vi "TcA02-003_ModifyingObjectAttributesMultipleTimes.vi"(1 "Input buffer":T3="1", 3 "Invocation info":T2, 5 "error in (no error)":errorcluster, 6 "Add log to result?":bool) -> (16 "Test Data":T1 {"Numeric Measurement" format="%.2f"}, 19 "error out":errorcluster)   [LabVIEW 2020]
doc: "Test case template."
uses:
  Shared/Support_InputBuffer.ctl
  Shared/Support_InvocationInfo.ctl
  Shared/Support_TestData.ctl
  TestClasses/G#SubClass2_class/G#SubClass2.lvclass
  TestClasses/G#BaseClass2_class/G#BaseClass2.lvclass
  TestClasses/G#BaseClass1_class/G#BaseClass1.lvclass
  <vilib>/addons/_AddQ/G#Object/G#Object.lvclass
panel:
  in  "Test name":string="TcA02-003 Modifying object attributes multiple times"
  out "Test result":bool
  out "Result":string
  # "Verify that object attributes can be modified\nmultiple times unaffected by other objects."
  # "Sub test case"
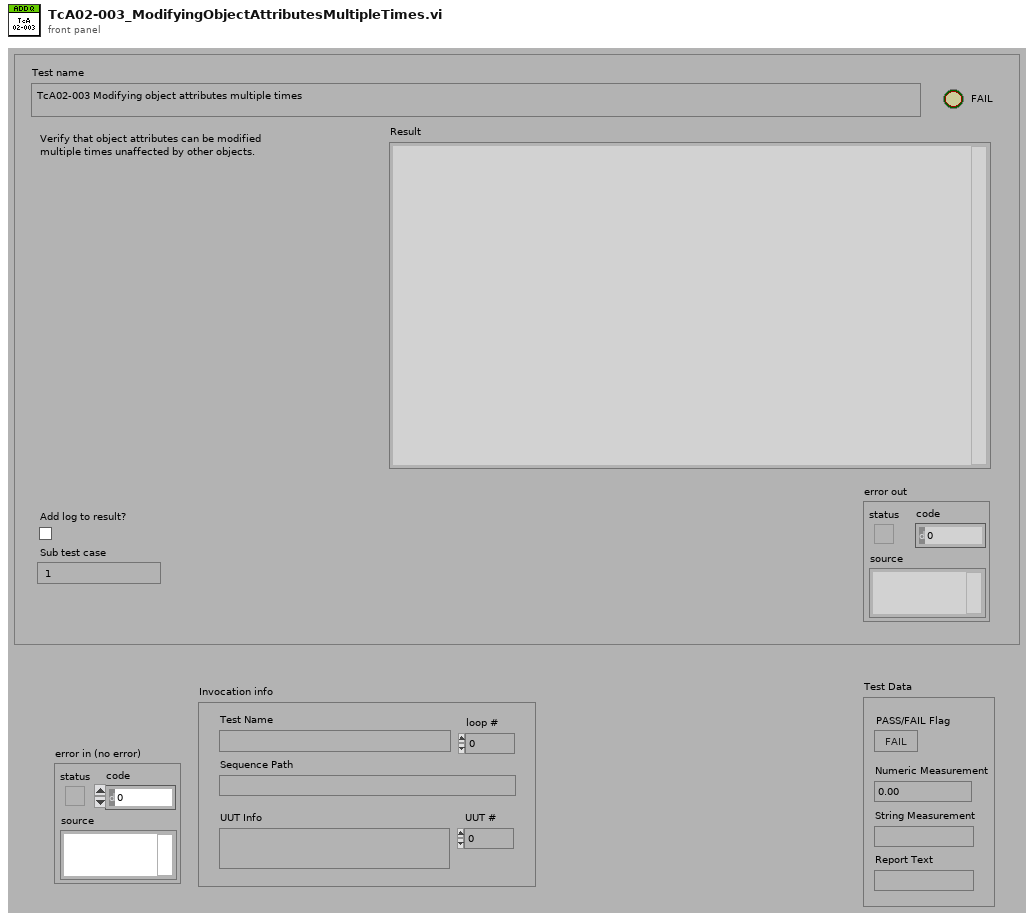
[diagram p1: front panel]
types:
  T1 = typedef "Support_TestData.ctl" = cluster{"PASS/FAIL Flag":bool, "Numeric Measurement":dbl, "String Measurement":string, "Report Text":string}
  T2 = typedef "Support_InvocationInfo.ctl" = cluster{"UUT #":i32, "loop #":i32, "UUT Info":string, "Test Name":string, "Sequence Path":path}
  T3 = typedef "Support_InputBuffer.ctl" = string
  T4 = typedef "Support_ResultType.ctl" = cluster{"Pass":bool, "Comment":string, "MeasurementValue":dbl}
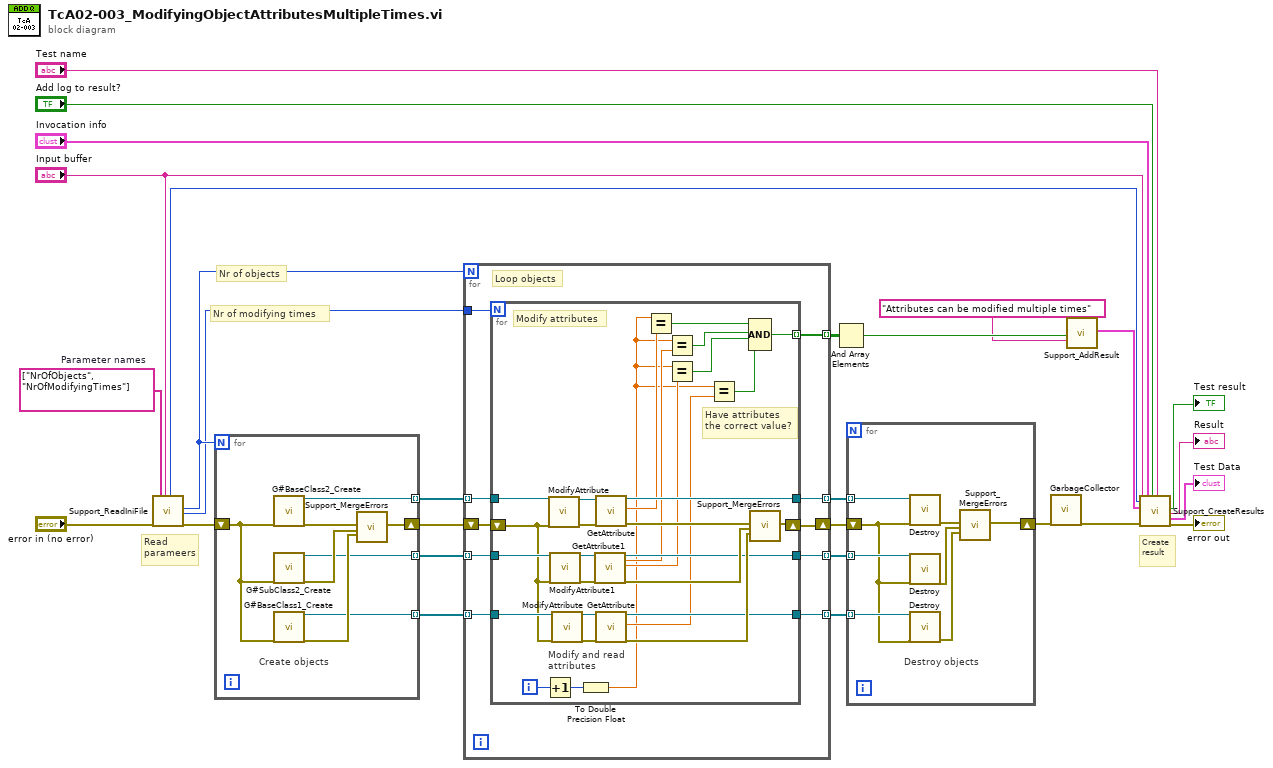
[diagram p0: block diagram]
diagram:
  w18 = string[] ["NrOfObjects", "NrOfModifyingTimes"]  # Parameter names
  # "Nr of modifying times"
  # "Nr of objects"
  # "Create\nresult"
  # "Read\nparameers"
  n1 = call "Support_ReadIniFile.vi"("error in (no error)"="error in (no error)", "Parameter names"=w18, "Sub test case"="Input buffer") -> ("Timer start"=w19:u32, "Parameter1 as I32"=w13:i32, "Parameter2 as I32"=w12:i32, "error out"=w17:errorcluster)  [unwired: 9 in, 4 out]
  n2 = for {
    N: w13 -> [_]
    shift-right: [w36] -> w11
    shift-left: w17 -> [w35]
    tunnel: [w31] -> w15 mode=indexing
    tunnel: [w30] -> w16 mode=indexing
    tunnel: [w29] -> w14 mode=indexing
    # "Create objects"
    n3 = call "G#BaseClass2_Create.vi"("error in (no error)"=w35) -> ("reference out"=w31:refnum<class "G#BaseClass2.lvclass">, "error out"=w34:errorcluster)  [unwired: 17 in]
    n4 = call "G#SubClass2_Create.vi"("error in (no error)"=w35) -> ("reference out"=w30:refnum<class "G#SubClass2.lvclass">, "error out"=w33:errorcluster)  [unwired: 17 in]
    n5 = call "G#BaseClass1_Create.vi"("error in (no error)"=w35) -> ("reference out"=w29:refnum<class "G#BaseClass1.lvclass">, "error out"=w32:errorcluster)  [unwired: 16 in, 1 out]
    n6 = call "Support_MergeErrors.vi"("error in 1"=w34, "error in 2"=w33, "error in 3"=w32) -> ("error out"=w36:errorcluster)  [unwired: 15 in, 1 out]
  }
  n7 = for {
    N: w13 -> [_]
    tunnel: w16 -> [w46] mode=indexing
    tunnel: w15 -> [w45] mode=indexing
    tunnel: w14 -> [w44] mode=indexing
    tunnel: w12 -> [w43]
    shift-right: [w41] -> w10
    shift-left: w11 -> [w42]
    tunnel: [w40] -> w9 mode=indexing
    tunnel: [w39] -> w8 mode=indexing
    tunnel: [w38] -> w7 mode=indexing
    tunnel: [w37] -> w4 mode=indexing
    # "Loop objects"
    n8 = for {
      N: w43 -> [_]
      shift-right: [w62] -> w41
      shift-left: w42 -> [w72]
      tunnel: w46 -> [w75]
      tunnel: w45 -> [w74]
      tunnel: w44 -> [w73]
      tunnel: [w61] -> w40
      tunnel: [w60] -> w39
      tunnel: [w59] -> w38
      tunnel: [w48] -> w37 mode=indexing
      i -> [w58]
      # "Modify and read\nattributes"
      # "Have attributes\nthe correct value?"
      # "Modify attributes"
      n9 = Increment(x=w58) -> (x+1=w54:i32)
      n10 = call-dynamic "ModifyAttribute.vi"("reference in"=w74, "error in (no error)"=w72) -> ("reference out"=w68:refnum<class "G#BaseClass2.lvclass">, "error out"=w69:errorcluster)  [unwired: 15 in, 1 out]
      n11 = call-dynamic "ModifyAttribute1.vi"("reference in"=w75, "error in (no error)"=w72) -> ("reference out"=w67:refnum<class "G#SubClass2.lvclass">, "error out"=w70:errorcluster)  [unwired: 15 in, 1 out]
      n12 = call-dynamic "ModifyAttribute.vi"("reference in"=w73, "error in (no error)"=w72) -> ("reference out"=w66:refnum<class "G#BaseClass1.lvclass">, "error out"=w71:errorcluster)  [unwired: 16 in]
      n13 = To Double Precision Float(number=w54) -> (double precision float=w47:dbl)
      n14 = call-dynamic "GetAttribute1.vi"("reference in"=w67, "error in (no error)"=w70) -> ("reference out"=w60:refnum<class "G#SubClass2.lvclass">, "Base class.Numeric"=w56:dbl, "SubAttribute"=w55:dbl, "error out"=w64:errorcluster)  [unwired: 12 in, 2 out]
      n15 = call-dynamic "GetAttribute.vi"("reference in"=w68, "error in (no error)"=w69) -> ("reference out"=w61:refnum<class "G#BaseClass2.lvclass">, "Numeric"=w57:dbl, "error out"=w65:errorcluster)  [unwired: 13 in, 2 out]
      n16 = call-dynamic "GetAttribute.vi"("reference in"=w66, "error in (no error)"=w71) -> ("reference out"=w59:refnum<class "G#BaseClass1.lvclass">, "Numeric"=w53:dbl, "error out"=w63:errorcluster)  [unwired: 14 in, 1 out]
      n17 = Equal?(x=w47, y=w57) -> (x = y?=w52:bool)
      n18 = Equal?(x=w47, y=w56) -> (x = y?=w51:bool)
      n19 = Equal?(x=w47, y=w55) -> (x = y?=w50:bool)
      n20 = Equal?(x=w47, y=w53) -> (x = y?=w49:bool)
      n21 = Compound Arithmetic op=AND(w52, w51, w50, w49) -> (w48:bool)
      n22 = call "Support_MergeErrors.vi"("error in 1"=w65, "error in 2"=w64, "error in 3"=w63) -> ("error out"=w62:errorcluster)  [unwired: 15 in, 1 out]
    }
  }
  n23 = And Array Elements(Boolean array=w4) -> (logical AND=w3:bool)
  n24 = for {
    shift-right: [w76] -> w6
    shift-left: w10 -> [w80]
    tunnel: w9 -> [w83] mode=indexing
    tunnel: w8 -> [w82] mode=indexing
    tunnel: w7 -> [w81] mode=indexing
    # "Destroy objects"
    n25 = call-dynamic "Destroy.vi"("reference in"=w83, "error in (no error)"=w80) -> ("error out"=w79:errorcluster)  [unwired: 16 in, 1 out]
    n26 = call-dynamic "Destroy.vi"("reference in"=w82, "error in (no error)"=w80) -> ("error out"=w78:errorcluster)  [unwired: 16 in, 1 out]
    n27 = call-dynamic "Destroy.vi"("reference in"=w81, "error in (no error)"=w80) -> ("error out"=w77:errorcluster)  [unwired: 16 in, 1 out]
    n28 = call "Support_MergeErrors.vi"("error in 1"=w79, "error in 2"=w78, "error in 3"=w77) -> ("error out"=w76:errorcluster)  [unwired: 15 in, 1 out]
  }
  n29 = call <vilib>:"GarbageCollector.vi"("error in (no error)"=w6) -> ("error out"=w5:errorcluster)  [unwired: 16 in, 2 out]
  n30 = call "Support_AddResult.vi"("Pass"=w3, "Comment"="Attributes can be modified multiple times") -> ("Results out"=w2:T4[])  [unwired: 17 in]
  n31 = call "Support_CreateResults.vi"("Sub test case"="Input buffer", "Timer start"=w19, "Results"=w2, "error in (no error)"=w5, "Invocation info"="Invocation info", "Add log to result?"="Add log to result?", "Test name"="Test name") -> ("Pass/fail flag"=→"Test result":bool, "Result"=→"Result":string, "Test Data"=→"Test Data":T1, "error out"=→"error out":errorcluster)  [unwired: 9 in]
